vi "Initialize.vi"(8 "error in":errorcluster, 10 "shared resources":refnum<class "Shared Resources.lvclass">, 11 "Tx Execution Unit Implementation in":refnum<class "Tx Execution Unit.lvclass">) -> (0 "error out":errorcluster, 3 "Tx Execution Unit Implementation out":refnum<class "Tx Execution Unit.lvclass">)   [LabVIEW 2020, in "Ballard MIL-STD-1553 Engine.lvlib" / "Implementation.lvlib" / "Tx Execution Unit.lvclass"]
uses:
  Tx Execution Unit.lvclass
  C:/dev/niveristand-ballard-milStd1553-custom-device/Source/Custom Device Support/Engine/Implementation/Execution Unit/Execution Unit.lvclass
  Interfaces/Shared Resources/Shared Resources.lvclass
  Execution Unit/Execution Unit.lvclass/Execution Unit.ctl
  Tx Execution Unit.lvclass/Tx Execution Unit.ctl
  Execution Unit/Execution Unit.lvclass
  Custom Device/Custom Device.lvlib
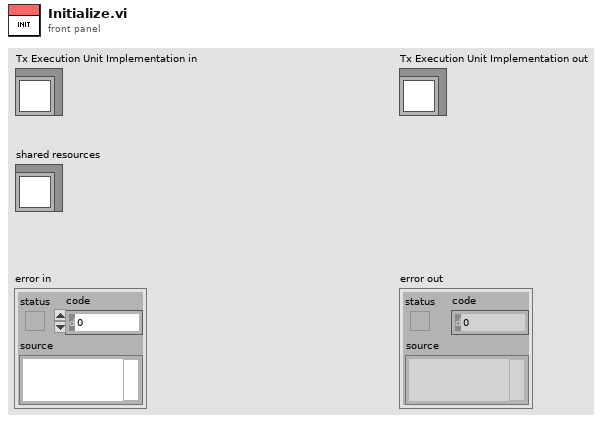
[diagram p1: front panel]
types:
  T1 = typedef "1553 Channel.ctl" = cluster{"HW channel":u16, "terminals":T2[], "messages":T4[], "acyclic frame names":string[]}
  T2 = typedef "Terminal Name and Address.ctl" = cluster{"name":string, "terminal address":T3}
  T3 = typedef "Address.ctl" = u16
  T4 = typedef "Message Definition.ctl" = cluster{"name":string, "message type":T5, "endpoint Rx":T6, "endpoint Tx":T6, "mode code":u16, "number of words":u16, "parameters":cluster{"name":string, "default value":dbl, "unit":string, "parameter definition":T7}[], "create timestamp channel":bool}
  T5 = typedef "Message Type.ctl" = string
  T6 = typedef "Terminal Endpoint.ctl" = cluster{"terminal address":T3, "subaddress":T3}
  T7 = typedef "Parameter Definition.ctl" = cluster{"start index":i32, "size (bits)":i32, "encoding":enum16{"BNR", "BCD", "Discrete"}, "signed":bool, "multiplier":dbl, "offset":dbl}
  T8 = typedef "Ballard MIL-STD-1553 Engine.lvlib/Custom Device.lvlib/Hardware Handles.ctl" = cluster{"core handle":u64, "core reader handle":u64, "channel handles":u64[]}
  T9 = typedef "Map of Message Indexes to Tx Write Info.ctl" = map{i32, T10}
  T10 = typedef "Tx Write Info.ctl" = cluster{"rt transfer handle":u64, "value index":i32}
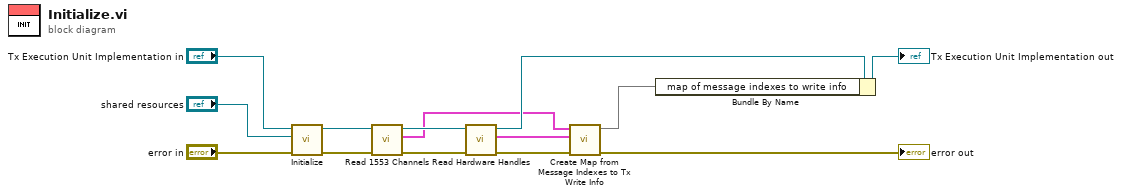
[diagram p0: block diagram]
diagram:
  n1 = call-parent "Initialize.vi"("error in"="error in", "shared resources"="shared resources", "Execution Unit Implementation in"="Tx Execution Unit Implementation in") -> ("error out"=w9:errorcluster, "Execution Unit Implementation out"=w11:refnum<class "Tx Execution Unit.lvclass">)  [unwired: 7 in]
  n2 = call "Read 1553 Channels.vi"("error in"=w9, "Execution Unit in"=w11) -> ("error out"=w7:errorcluster, "1553 channels"=w2:T1[], "Execution Unit out"=w5:refnum<class "Tx Execution Unit.lvclass">)  [unwired: 7 in]
  n3 = call "Read Hardware Handles.vi"("error in"=w7, "Execution Unit in"=w5) -> ("error out"=w6:errorcluster, "hardware handles"=w3:T8, "Execution Unit out"=w4:refnum<class "Tx Execution Unit.lvclass">)  [unwired: 7 in]
  n4 = call "Create Map from Message Indexes to Tx Write Info.vi"("error in"=w6, "hardware handles"=w3, "1553 channels"=w2) -> ("error out"=→"error out":errorcluster, "map from message indexes to Tx write info"=w1:T9)  [unwired: 7 in]
  n5 = Bundle By Name(cluster=w4, "map of message indexes to write info"=w1) -> (→"Tx Execution Unit Implementation out":refnum<class "Tx Execution Unit.lvclass">)
